vi "Modbus Write U8.vi"(7 "Slave Address":u8, 8 "error in (no error)":errorcluster, 9 "Input data U8":u8, 10 "Register Start Address":u16 format="%x", 11 "VISA resource in":refnum<visa-resource-name>) -> (0 "error out":errorcluster, 3 "VISA resource out":refnum<visa-resource-name>)   [LabVIEW 2023, in "Voegtlin_NI_SMART_Modbus_Drivers.lvlib"]
doc: "Schreibe einen U8-Wert an die angegebene Startadresse des selektierten Geraetes. Es wird ein Register geschrieben, wobei das high-Byte leer bleibt.\nDer COM-Port muss dazu initialisiert sein (benutze\" Modbus Init.vi\")."
uses:
  Voegtlin_NI_SMART_Modbus_Drivers.lvlib
  Enums/Modbus Comm.ctl
panel:
  out "U16 input data to write\n(array)":u16[](array[numeric])
  # "Input Data"
  # "Internal Data"
  # "Output Data"
  # "(Inputmaske in HEX)"
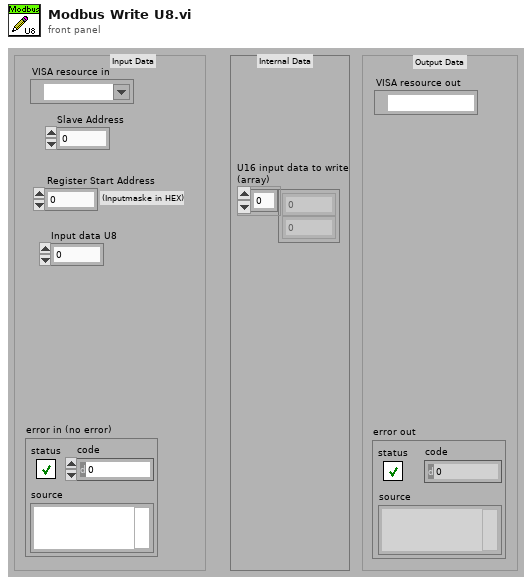
[diagram p1: front panel]
types:
  T1 = typedef "Voegtlin_NI_SMART_Modbus_Drivers.lvlib/Modbus Comm.ctl" = enum16{"Init", "Read", "Write", "Exit"}
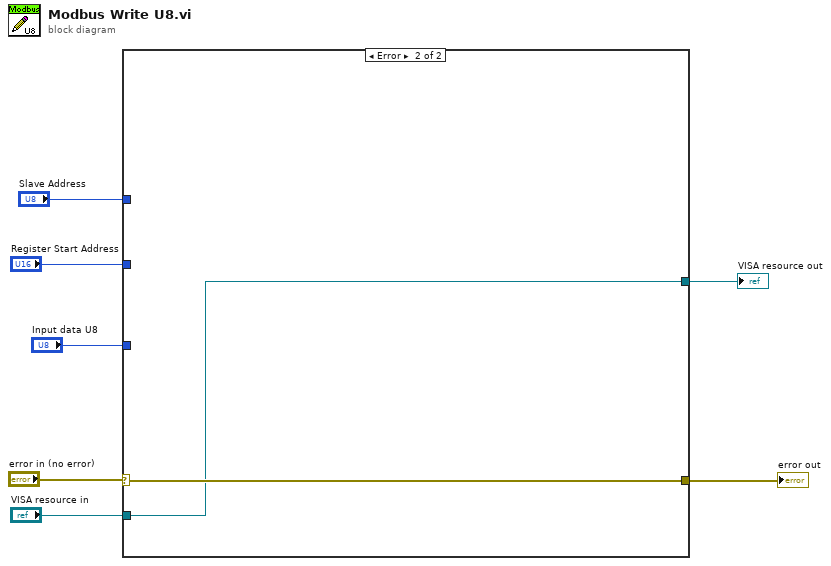
[diagram p0: block diagram]
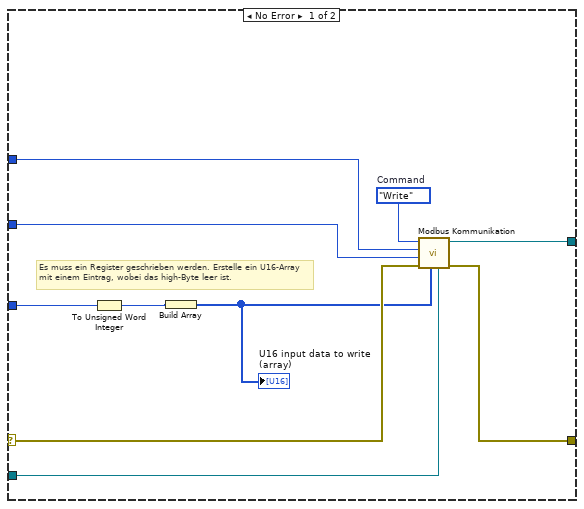
[diagram p2: hidden frame]
diagram:
  n1 = case shown="Error" "error in (no error)" {
    selector: "error in (no error)" -> [w13 w19]
    tunnel: "Register Start Address" -> [w12 _]
    tunnel: [w17 w19] -> w6
    tunnel: "Input data U8" -> [w15 _]
    tunnel: "Slave Address" -> [w10 _]
    tunnel: [w9 w18] -> w2
    tunnel: "VISA resource in" -> [w8 w18]
    frame No Error {
      w16 = Modbus_Comm."Write"  # Command
      # "Es muss ein Register geschrieben werden. Erstelle ein U16-Array mit einem Eintrag, wobei das high-Byte leer ist."
      n2 = To Unsigned Word Integer(number=w15) -> (unsigned 16bit integer=w14:u16)
      n3 = Build Array(w14) -> (w11:u16[])
      "U16 input data to write\n(array)" <- w11
      n4 = call "Modbus Kommunikation.vi"("VISA resource in"=w8, "Data In / #Reads [U16]"=w11, "error in (no error)"=w13, "Register Start Address"=w12, "Slave Address"=w10, "Command"=w16) -> ("error out"=w17:errorcluster, "VISA resource out"=w9:refnum<visa-resource-name>)  [unwired: 3 in, 1 out]
    }
    frame Error {
    }
  }
  "error out" <- w6
  "VISA resource out" <- w2
